vi "Harvester_1_26.vi"() -> ()   [LabVIEW 2013]
panel:
  out "HarvRoller":dbl
  out "HarvPower":dbl
  in  "LimitSwitchIn":bool
  in  "LimitSwitchOut":bool
  in  "InButton":bool
  in  "OutButton":bool
  in  "HarvInPos":dbl
  in  "HarvOutPos":dbl
  in  "HarvPot":dbl
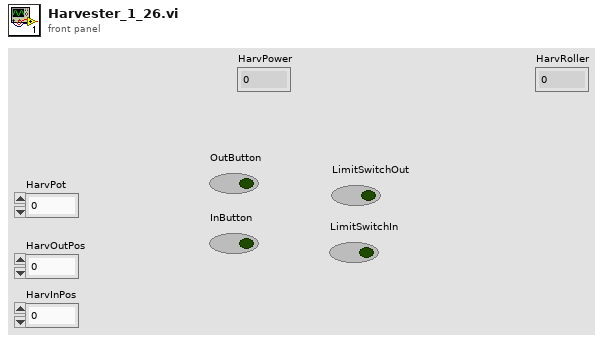
[diagram p1: front panel]
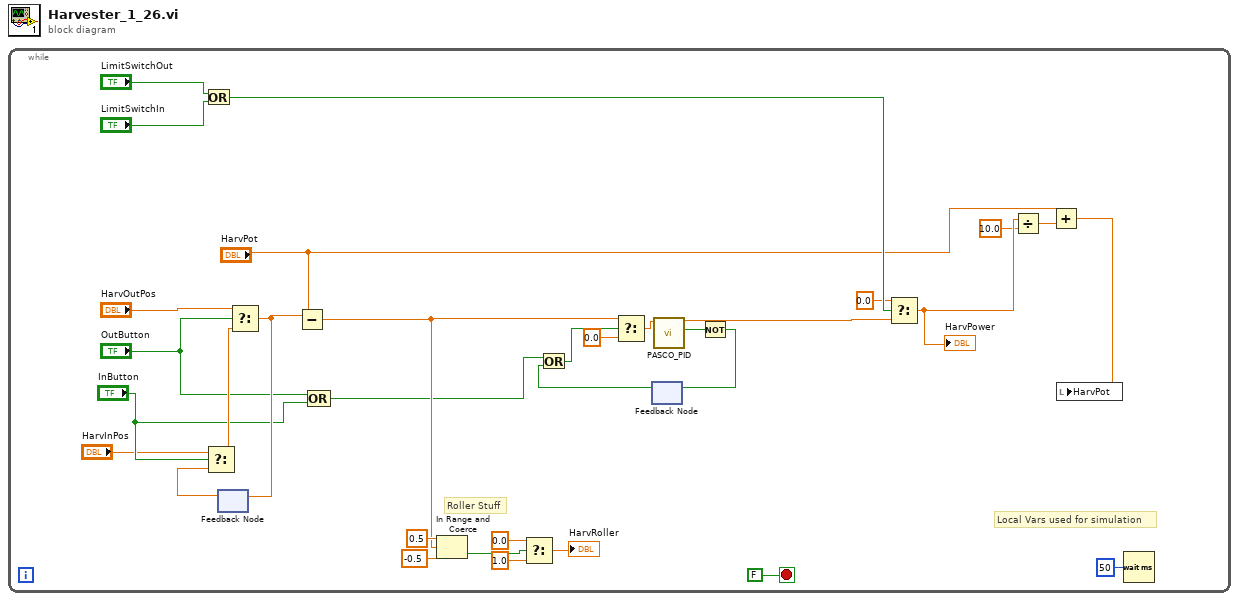
[diagram p0: block diagram]
diagram:
  n1 = while {
    stop <- FALSE stop-if-true
    # "Roller Stuff"
    # "Local Vars used for simulation"
    n2 = Or(x="LimitSwitchOut", y="LimitSwitchIn") -> (x .or. y?=w22:bool)
    n3 = feedback #1() -> (w31:dbl)  [unwired: 1 in]
    n4 = Select(t="HarvInPos", s="InButton", f=w31) -> (s? t:f=w32:dbl)
    n5 = Select(t="HarvOutPos", s="OutButton", f=w32) -> (s? t:f=w30:dbl)
    n6 = feedback-in #1(w30) -> ()
    n7 = Subtract(x=w30, y="HarvPot") -> (x-y=w7:dbl)
    n8 = Compound Arithmetic op=OR("OutButton", "InButton") -> (w4:bool)
    n9 = In Range and Coerce(upper limit=0.5, x=w7, lower limit=-0.5) -> (In Range?=w11:bool)  [unwired: 1 out]
    n10 = Select(t=0.0, s=w11, f=1.0) -> (s? t:f=→"HarvRoller":dbl)
    n11 = feedback #2() -> (w2:bool)  [unwired: 1 in]
    n12 = Or(x=w4, y=w2) -> (x .or. y?=w3:bool)
    n13 = Select(t=w7, s=w3, f=0.0) -> (s? t:f=w24:dbl)
    n14 = call "PASCO_PID.vi"("Delta"=w24) -> ("Power Out"=w21:dbl, "IsThere"=w25:bool)  [unwired: 13 in]
    n15 = Not(x=w25) -> (.not. x?=w23:bool)
    n16 = feedback-in #2(w23) -> ()
    n17 = Select(t=0.0, s=w22, f=w21) -> (s? t:f=w18:dbl)
    "HarvPower" <- w18
    n18 = Divide(x=w18, y=10.0) -> (x/y=w6:dbl)
    n19 = Add(x="HarvPot", y=w6) -> (x+y=w17:dbl)
    n20 = local write "HarvPot"(w17) -> ()
    n21 = Wait (ms)(milliseconds to wait=u32 50) -> ()  [unwired: 1 out]
  }
